vi "Lookup Sensor Scale.vi"(7 "SensorList":refnum<class "SensorList.lvclass">, 8 "error in (no error)":errorcluster, 11 "Scale in":refnum<class "Scale.lvclass">) -> (0 "error out":errorcluster, 2 "Sensor Scale":refnum<class "Scale.lvclass">, 3 "Scale out":refnum<class "Scale.lvclass">)   [LabVIEW 2020, in "VolatusConfig.lvlib" / "Scale.lvclass"]
uses:
  Scale.lvclass
  C:/dev/lv20CE/relink/lv-volatus/VolatusConfig/VolatusConfigElement/VolatusConfigElement.lvclass
  SensorList/SensorList.lvclass
  VolatusConfigElement/VolatusConfigElement.lvclass/VolatusConfigElement.ctl
  Meta Type.ctl
  VolatusConfigElement/Element.vi
  lv-cdm/CDM-Config/Config Lookup/Match Meta.vi
  lv-cdm/CDM-Config/Config Element/Owner.vi
  lv-cdm/CDM-Config/Config Manager/Lookup Descendant.vi
  lv-cdm/CDM-Config/Config Filter/Config Lookup.lvclass
  Scale.lvclass/Scale.ctl
  VolatusConfigElement/VolatusConfigElement.lvclass
  VolatusConfig.lvlib
  lv-cdm/CDM-Config/Config Element/Config Element.lvclass
  Sensor/Sensor.lvclass
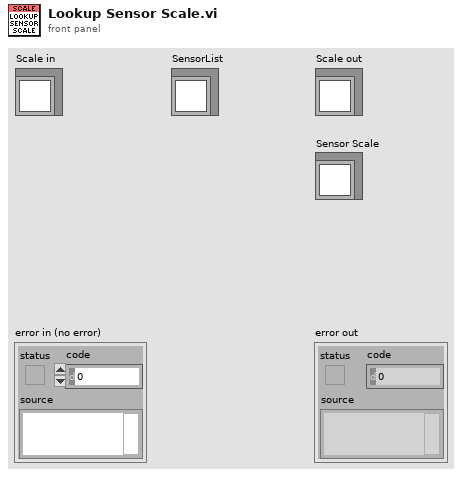
[diagram p1: front panel]
types:
  T1 = typedef "VolatusConfig.lvlib/Meta Type.ctl" = enum16{"UNKNOWN", "VL_System", "VL_Cluster", "VL_Node", "VL_Task", "VL_Group", "VL_Channel", "VL_Task_List", "VL_Scaling", "VL_Sensor", "VL_Sensor_List", "VL_Scale"}
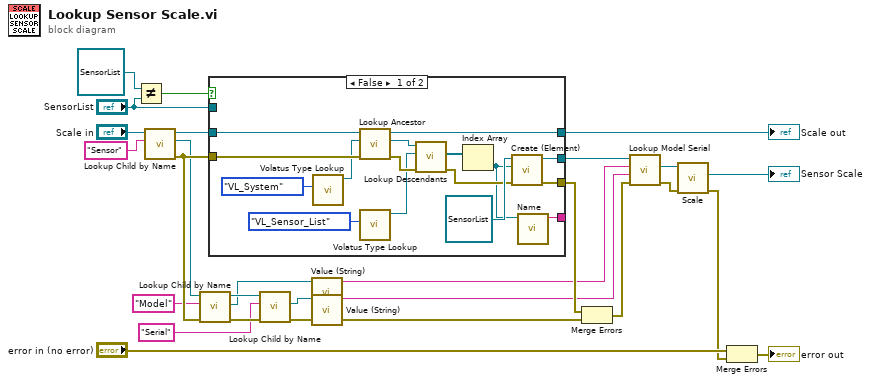
[diagram p0: block diagram]
diagram:
  n1 = Not Equal?(x=refnum<class "SensorList.lvclass"> refnum, y="SensorList") -> (x != y?=w3:bool)
  n2 = call "Lookup Child by Name.vi"("Child Name"="Sensor", "VolatusConfigElement in"="Scale in") -> ("error out"=w26:errorcluster, "Child"=w22:refnum<class "Config Element.lvclass">, "VolatusConfigElement out"=w24:refnum<class "Scale.lvclass">)  [unwired: 6 in, 1 out]
  n3 = call "Lookup Child by Name.vi"("error in (no error)"=w26, "Name"="Model", "Config Element in"=w22) -> ("error out"=w19:errorcluster, "Child"=w17:refnum<class "Config Element.lvclass">, "Config Element out"=w20:refnum<class "Config Element.lvclass">)  [unwired: 5 in, 1 out]
  n4 = case shown="False" w3 {
    tunnel: w26 -> [w43 w44]
    tunnel: w24 -> [w35 w46]
    tunnel: [w33 w46] -> w14
    tunnel: [w32 w45] -> w13
    tunnel: "SensorList" -> [_ w45]
    tunnel: [w30 w44] -> w27
    tunnel: [w28 _] -> _
    frame False {
      n5 = call "Volatus Type Lookup.vi"("Meta Type"=Meta_Type."VL_System") -> ("Config Lookup out"=w41:refnum<class "Config Lookup.lvclass">)  [unwired: 9 in, 1 out]
      n6 = call "Lookup Ancestor.vi"("error in (no error)"=w43, "Lookup"=w41, "VolatusConfigElement in"=w35) -> ("error out"=w42:errorcluster, "Ancestor"=w39:refnum<class "Config Element.lvclass">, "VolatusConfigElement out"=w33:refnum<class "Scale.lvclass">)  [unwired: 6 in]
      n7 = call "Volatus Type Lookup.vi"("Meta Type"=Meta_Type."VL_Sensor_List") -> ("Config Lookup out"=w37:refnum<class "Config Lookup.lvclass">)  [unwired: 9 in, 1 out]
      n8 = call "Lookup Descendants.vi"("error in (no error)"=w42, "Lookup"=w37, "Config Element in"=w39) -> ("error out"=w31:errorcluster, "Descendants"=w36:refnum<class "Config Element.lvclass">[])  [unwired: 6 in, 1 out]
      n9 = Index Array(array=w36) -> (element=w29:refnum<class "Config Element.lvclass">)  [unwired: 1 in]
      n10 = call "Create (Element).vi"("error in (no error)"=w31, "Element"=w29, "VolatusConfigElement in"=refnum<class "SensorList.lvclass"> refnum ("VolatusConfig.lvlib:SensorList.lvclass")) -> ("error out"=w30:errorcluster, "VolatusConfigElement out"=w32:refnum<class "SensorList.lvclass">)  [unwired: 7 in]
      n11 = call "Name.vi"("Config Element in"=w29) -> ("Name"=w28:string)  [unwired: 9 in, 1 out]
    }
    frame True {
    }
  }
  "Scale out" <- w14
  n12 = call "Lookup Child by Name.vi"("error in (no error)"=w19, "Name"="Serial", "Config Element in"=w20) -> ("error out"=w15:errorcluster, "Child"=w16:refnum<class "Config Element.lvclass">)  [unwired: 5 in, 2 out]
  n13 = call "Value (String).vi"("Config Element in"=w17) -> ("String Value"=w12:string)  [unwired: 9 in, 1 out]
  n14 = call "Value (String).vi"("Config Element in"=w16) -> ("String Value"=w11:string)  [unwired: 9 in, 1 out]
  n15 = Merge Errors(w27, w15) -> (w1:errorcluster)
  n16 = call "Lookup Model Serial.vi"("error in (no error)"=w1, "Serial"=w11, "Model"=w12, "SensorList in"=w13) -> ("error out"=w9:errorcluster, "Sensor"=w10:refnum<class "Sensor.lvclass">)  [unwired: 5 in, 1 out]
  n17 = call "Scale.vi"("error in (no error)"=w9, "Sensor in"=w10) -> ("error out"=w6:errorcluster, "Sensor Scale"=→"Sensor Scale":refnum<class "Scale.lvclass">)  [unwired: 7 in, 1 out]
  n18 = Merge Errors("error in (no error)", w6) -> (→"error out":errorcluster)
